vi "Close DB.vi"(8 "error in (no error)":errorcluster, 11 "DataBase_SQL in":refnum<class "DataBase_SQL.lvclass">) -> (0 "error out":errorcluster, 3 "DataBase_SQL out":refnum<class "DataBase_SQL.lvclass">)   [LabVIEW 2021, in "DataBase_SQL.lvclass"]
uses:
  <userlib>/John_Lib/DataBase/DataBase_SQL/DataBase_SQL.lvclass
  <userlib>/John_Lib/DataBase/DataBase_SQL/DataBase_SQL.lvclass/DataBase_SQL.ctl
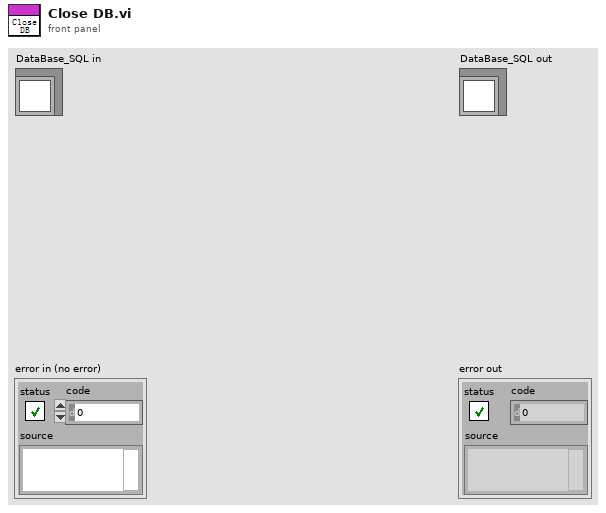
[diagram p1: front panel]
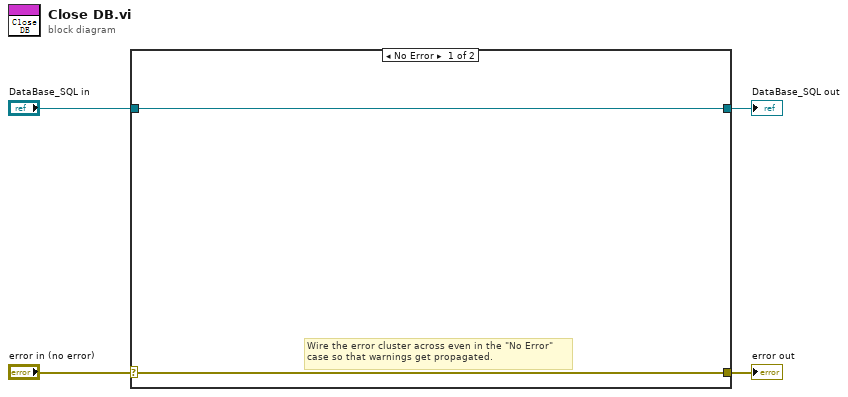
[diagram p0: block diagram]
diagram:
  n1 = case shown="No Error" "error in (no error)" {
    selector: "error in (no error)" -> [w5 w8]
    tunnel: [w5 w8] -> w3
    tunnel: [w6 w7] -> w1
    tunnel: "DataBase_SQL in" -> [w6 w7]
    frame No Error {
      # "Wire the error cluster across even in the \"No Error\"\ncase so that warnings get propagated."
    }
    frame Error {
    }
  }
  "error out" <- w3
  "DataBase_SQL out" <- w1
